vi "simulated_scope_mss_test1.vi"(8 "Error In":errorcluster) -> (0 "Error Out":errorcluster)   [LabVIEW 2023]
uses:
  Measure and Stimulus Subsystems/Measure and Stimulus Subsystems.lvclass
panel:
  out "Powersensor Chart":waveform(dbl)(graph)
  in  "Stop":bool
  out "Photosensor Chart":waveform(dbl)(graph)
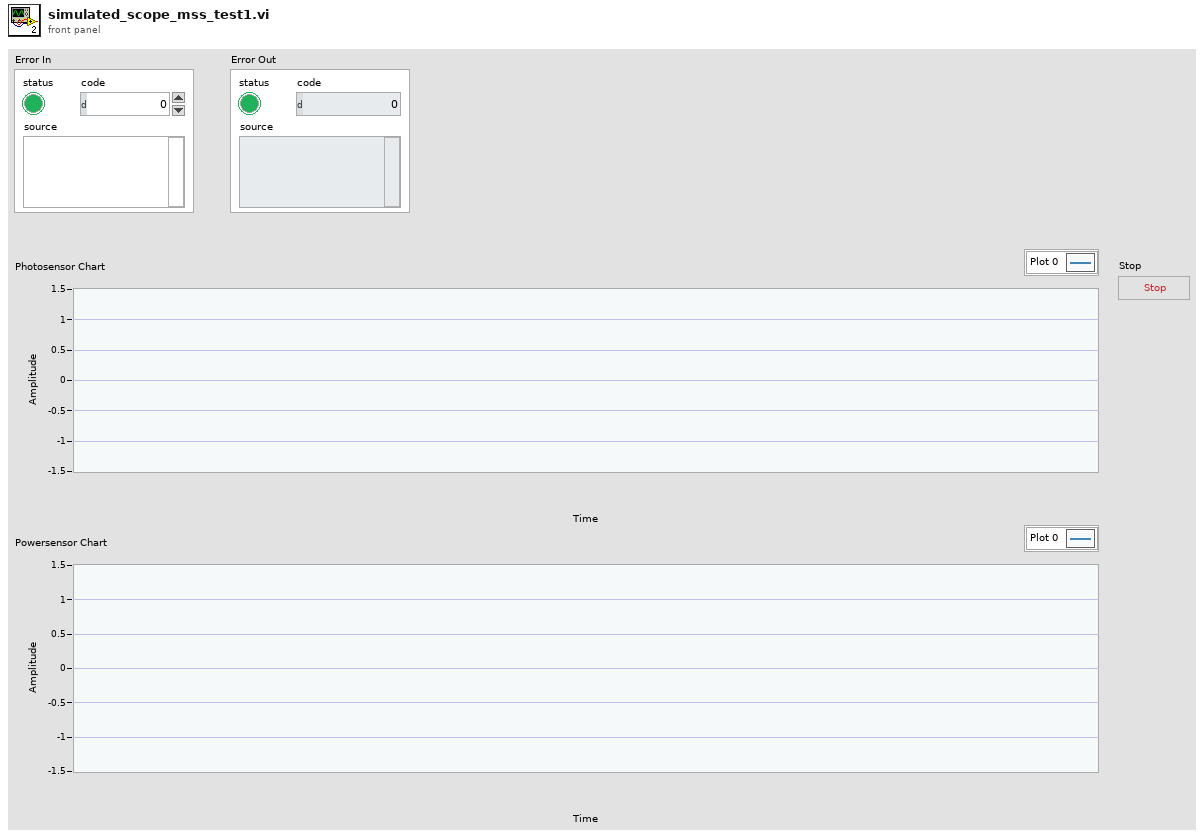
[diagram p1: front panel]
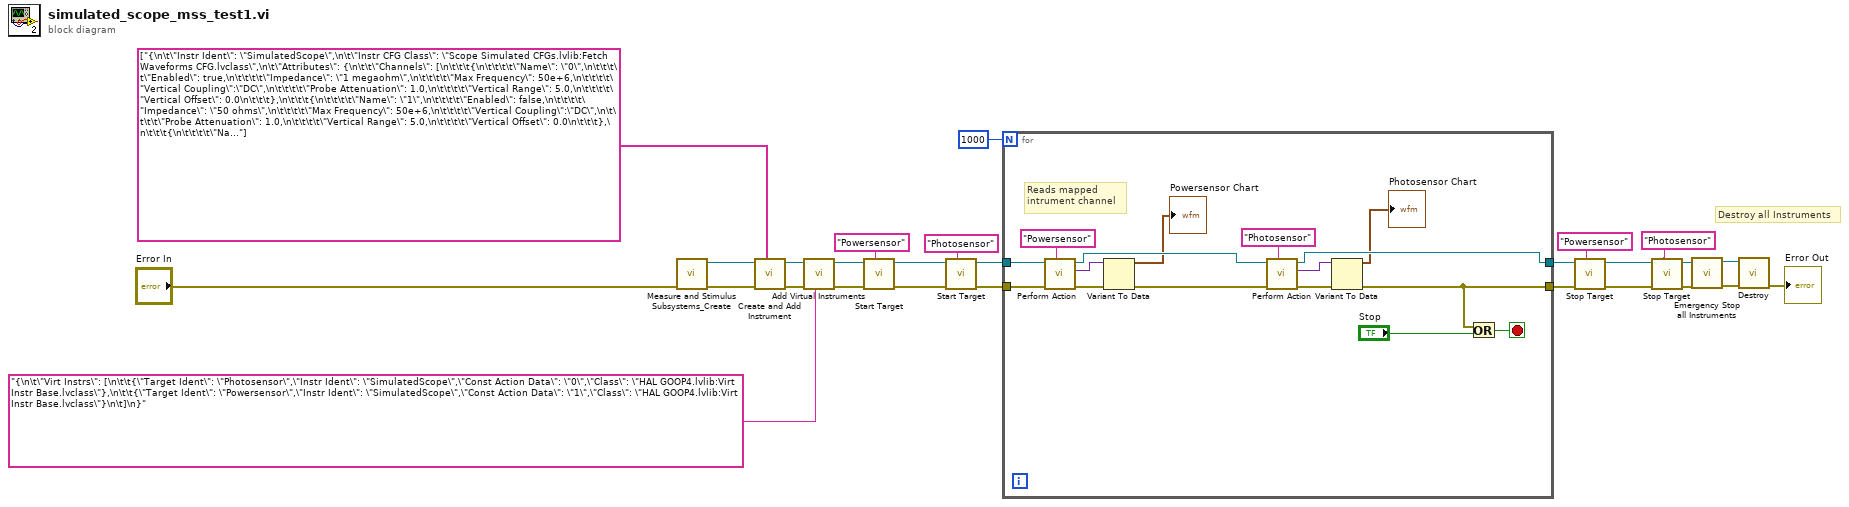
[diagram p0: block diagram]
diagram:
  # "Destroy all Instruments"
  n1 = call "Measure and Stimulus Subsystems_Create.vi"("Error In"="Error In") -> ("Error Out"=w26:errorcluster, "reference out"=w27:refnum<class "Measure and Stimulus Subsystems.lvclass">)  [unwired: 9 in]
  n2 = call "Create and Add Instrument.vi"("Physical Intr Configs"=string[] ["{\n\t\"Instr Ident\": \"SimulatedScope\",\n\t\"Instr CFG Class\": \"Scope Simulated CFGs.lvlib:Fetch Waveforms CFG.lvclass\",\n\t\"Attributes\": {\n\t\t\"Channels\": [\n\t\t\t{\n\t\t\t\t\"Name\": \"0\",\n\t\t\t\t\"Enabled\": true,\n\t\t\t\t\"Impedance\": \"1 megaohm\",\n\t\t\t\t\"Max Frequency\": 50e+6,\n\t\t\t\t\"Vertical Coupling\":\"DC\",\n\t\t\t\t\"Probe Attenuation\": 1.0,\n\t\t\t\t\"Vertical Range\": 5.0,\n\t\t\t\t\"Vertical Offset\": 0.0\n\t\t\t},\n\t\t\t{\n\t\t\t\t\"Name\": \"1\",\n\t\t\t\t\"Enabled\": false,\n\t\t\t\t\"Impedance\": \"50 ohms\",\n\t\t\t\t\"Max Frequency\": 50e+6,\n\t\t\t\t\"Vertical Coupling\":\"DC\",\n\t\t\t\t\"Probe Attenuation\": 1.0,\n\t\t\t\t\"Vertical Range\": 5.0,\n\t\t\t\t\"Vertical Offset\": 0.0\n\t\t\t},\n\t\t\t{\n\t\t\t\t\"Name\": \"2\",\n\t\t\t\t\"Enabled\": false,\n\t\t\t\t\"Impedance\": \"50 ohms\",\n\t\t\t\t\"Max Frequency\": 50e+6,\n\t\t\t\t\"Vertical Coupling\":\"DC\",\n\t\t\t\t\"Probe Attenuation\": 1.0,\n\t\t\t\t\"Vertical Range\": 5.0,\n\t\t\t\t\"Vertical Offset\": 0.0\n\t\t\t},\n\t\t\t{\n\t\t\t\t\"Name\": \"3\",\n\t\t\t\t\"Enabled\": true,\n\t\t\t\t\"Impedance\": \"50 ohms\",\n\t\t\t\t\"Max Frequency\": 50e+6,\n\t\t\t\t\"Vertical Coupling\":\"DC\",\n\t\t\t\t\"Probe Attenuation\": 1.0,\n\t\t\t\t\"Vertical Range\": 1.4,\n\t\t\t\t\"Vertical Offset\": 0.0\n\t\t\t},\n\t\t\t{\n\t\t\t\t\"Name\": \"4\",\n\t\t\t\t\"Enabled\": false,\n\t\t\t\t\"Impedance\": \"50 ohms\",\n\t\t\t\t\"Max Frequency\": 50e+6,\n\t\t\t\t\"Vertical Coupling\":\"DC\",\n\t\t\t\t\"Probe Attenuation\": 1.0,\n\t\t\t\t\"Vertical Range\": 5.0,\n\t\t\t\t\"Vertical Offset\": 0.0\n\t\t\t},\n\t\t\t{\n\t\t\t\t\"Name\": \"5\",\n\t\t\t\t\"Enabled\": false,\n\t\t\t\t\"Impedance\": \"50 ohms\",\n\t\t\t\t\"Max Frequency\": 50e+6,\n\t\t\t\t\"Vertical Coupling\":\"DC\",\n\t\t\t\t\"Probe Attenuation\": 1.0,\n\t\t\t\t\"Vertical Range\": 5.0,\n\t\t\t\t\"Vertical Offset\": 0.0\n\t\t\t},\n\t\t\t{\n\t\t\t\t\"Name\": \"6\",\n\t\t\t\t\"Enabled\": false,\n\t\t\t\t\"Impedance\": \"50 ohms\",\n\t\t\t\t\"Max Frequency\": 50e+6,\n\t\t\t\t\"Vertical Coupling\":\"DC\",\n\t\t\t\t\"Probe Attenuation\": 1.0,\n\t\t\t\t\"Vertical Range\": 5.0,\n\t\t\t\t\"Vertical Offset\": 0.0\n\t\t\t},\n\t\t\t{\n\t\t\t\t\"Name\": \"7\",\n\t\t\t\t\"Enabled\": false,\n\t\t\t\t\"Impedance\": \"50 ohms\",\n\t\t\t\t\"Max Frequency\": 50e+6,\n\t\t\t\t\"Vertical Coupling\":\"DC\",\n\t\t\t\t\"Probe Attenuation\": 1.0,\n\t\t\t\t\"Vertical Range\": 5.0,\n\t\t\t\t\"Vertical Offset\": 0.0\n\t\t\t}\n\t\t],\n\t\t\"Horizontal\": {\n\t\t\t\"Enforce Realtime\": true,\n\t\t\t\"Number of Records\": 1,\n\t\t\t\"Min Sample Rate\": 1e+5,\n\t\t\t\"Reference Position\":50, //percent\n\t\t\t\"Min Record Length\":1e+3\n\t\t},\n\t\t\"Acquire\": {\n\t\t\t\"Type\": \"Normal\",\n\t\t\t\"NumSamples\": 1e+3,\n\t\t\t\"Fetch Relative To\": \"Read Pointer\"\n\t\t},\n\t\t\"Export Signal\": {\n\t\t\t\"Signal Identifier\": \"None\",\n\t\t\t\"Signal\": \"None\",\n\t\t\t\"Output Terminal\": \"None\"\n\t\t},\n\t\t\"Trigger\": {\n\t\t\t\"Type\": \"Immediate\",\n\t\t\t\"Slope\": \"Positive\",\n\t\t\t\"Source\": \"RTSI 0\",\n\t\t\t\"Holdoff\": 0.0,\n\t\t\t\"Delay\": 0.0\n\t\t}\n\t}\n}"], "Error In"=w26, "reference in"=w27) -> ("Error Out"=w20:errorcluster, "reference out"=w3:refnum<class "Measure and Stimulus Subsystems.lvclass">)  [unwired: 7 in]
  n3 = call "Add Virtual Instruments.vi"("<JSON CFG>"="{\n\t\"Virt Instrs\": [\n\t\t{\"Target Ident\": \"Photosensor\",\"Instr Ident\": \"SimulatedScope\",\"Const Action Data\": \"0\",\"Class\": \"HAL GOOP4.lvlib:Virt Instr Base.lvclass\"},\n\t\t{\"Target Ident\": \"Powersensor\",\"Instr Ident\": \"SimulatedScope\",\"Const Action Data\": \"1\",\"Class\": \"HAL GOOP4.lvlib:Virt Instr Base.lvclass\"}\n\t]\n}", "Error In"=w20, "reference in"=w3) -> ("Error Out"=w4:errorcluster, "reference out"=w2:refnum<class "Measure and Stimulus Subsystems.lvclass">)  [unwired: 7 in]
  n4 = call "Start Target.vi"("Target Ident"="Powersensor", "Error In"=w4, "reference in"=w2) -> ("Error Out"=w18:errorcluster, "reference out"=w16:refnum<class "Measure and Stimulus Subsystems.lvclass">)  [unwired: 7 in]
  n5 = call "Start Target.vi"("Target Ident"="Photosensor", "Error In"=w18, "reference in"=w16) -> ("Error Out"=w17:errorcluster, "reference out"=w15:refnum<class "Measure and Stimulus Subsystems.lvclass">)  [unwired: 7 in]
  n6 = for {
    N: 1000 -> [_]
    tunnel: w17 -> [w36]
    tunnel: w15 -> [w35]
    tunnel: [w37] -> w11
    tunnel: [w39] -> w24
    stop <- w43 stop-if-true
    # "Reads mapped\nintrument channel"
    n7 = call "Perform Action.vi"("Target Ident"="Powersensor" ("Target Identifier"), "Error In"=w36, "reference in"=w35) -> ("Error Out"=w34:errorcluster, "Output"=w30:variant, "reference out"=w31:refnum<class "Measure and Stimulus Subsystems.lvclass">)  [unwired: 6 in]
    n8 = Variant To Data(error in=w34, Variant=w30) -> (data=→"Powersensor Chart":waveform(dbl), error out=w32:errorcluster)  [unwired: 1 in]
    n9 = call "Perform Action.vi"("Target Ident"="Photosensor" ("Target Identifier"), "Error In"=w32, "reference in"=w31) -> ("Error Out"=w41:errorcluster, "Output"=w38:variant, "reference out"=w37:refnum<class "Measure and Stimulus Subsystems.lvclass">)  [unwired: 6 in]
    n10 = Variant To Data(error in=w41, Variant=w38) -> (data=→"Photosensor Chart":waveform(dbl), error out=w39:errorcluster)  [unwired: 1 in]
    n11 = Or(x=w39, y="Stop") -> (x .or. y?=w43:bool)
  }
  n12 = call "Stop Target.vi"("Target Ident"="Powersensor", "Error In"=w24, "reference in"=w11) -> ("Error Out"=w12:errorcluster, "reference out"=w9:refnum<class "Measure and Stimulus Subsystems.lvclass">)  [unwired: 7 in]
  n13 = call "Stop Target.vi"("Target Ident"="Photosensor", "Error In"=w12, "reference in"=w9) -> ("Error Out"=w10:errorcluster, "reference out"=w8:refnum<class "Measure and Stimulus Subsystems.lvclass">)  [unwired: 7 in]
  n14 = call "Emergency Stop all Instruments.vi"("Error In"=w10, "reference in"=w8) -> ("Error Out"=w23:errorcluster, "reference out"=w22:refnum<class "Measure and Stimulus Subsystems.lvclass">)  [unwired: 8 in]
  n15 = call "Destroy.vi"("Error In"=w23, "reference in"=w22) -> ("Error Out"=→"Error Out":errorcluster)  [unwired: 8 in, 1 out]
